vi "FlyWheelSim_GetCurrentDrawAmps.vi"(11 "FlyWheelSim":T1 {"GearBox"."Jr_KgM2" format="%13.5p"; "GearBox"."L_H" format="%13.5p"; "GearBox"."Kt_NMPerAmp" format="%13.5p"; "GearBox"."KvINV_RadPerSecPerVolt" format="%13.5p"; "GearBox"."R_Ohms" format="%13.5p"; "GearBox"."FreeSpeed_RadPerSec" format="%13.5p"; "GearBox"."FreeCurrent_Amps" format="%13.5p"; "GearBox"."StallCurrent_Amps" format="%13.5p"; "GearBox"."StallTorque_NM" format="%13.5p"; "GearBox"."nominalVoltage_Volts" format="%13.5p"}) -> (3 "Current_Amps":dbl)   [LabVIEW 2019, in "Trajectory_Library.lvlib"]
doc: "Returns the flywheel current draw.\n\nInputs:\n - FlyWheelSim -- Data cluster\n \nOutputs:\n - Current_Amps -- The flywheel current draw. (Amps)"
uses:
  Trajectory_Library.lvlib
  FLYWHEEL_SIM.ctl
  LINEAR_SYSTEM_SIM.ctl
  LINEAR_SYSTEM.ctl
  <vilib>/Analysis/Matrix/Datatypes/RealMatrix.ctl
  DCMOTOR.CTL
  <vilib>/Analysis/Matrix/NI_Matrix.lvlib
panel:
  # "<States, 1>"
  # "<Outputs, 1>"
  # "<Inputs, 1>"
  # "<Outputs, 1>"
  # "<States,States>"
  # "<States,Inputs>"
  # "<Outputs,States>"
  # "<Outputs,Inputs>"
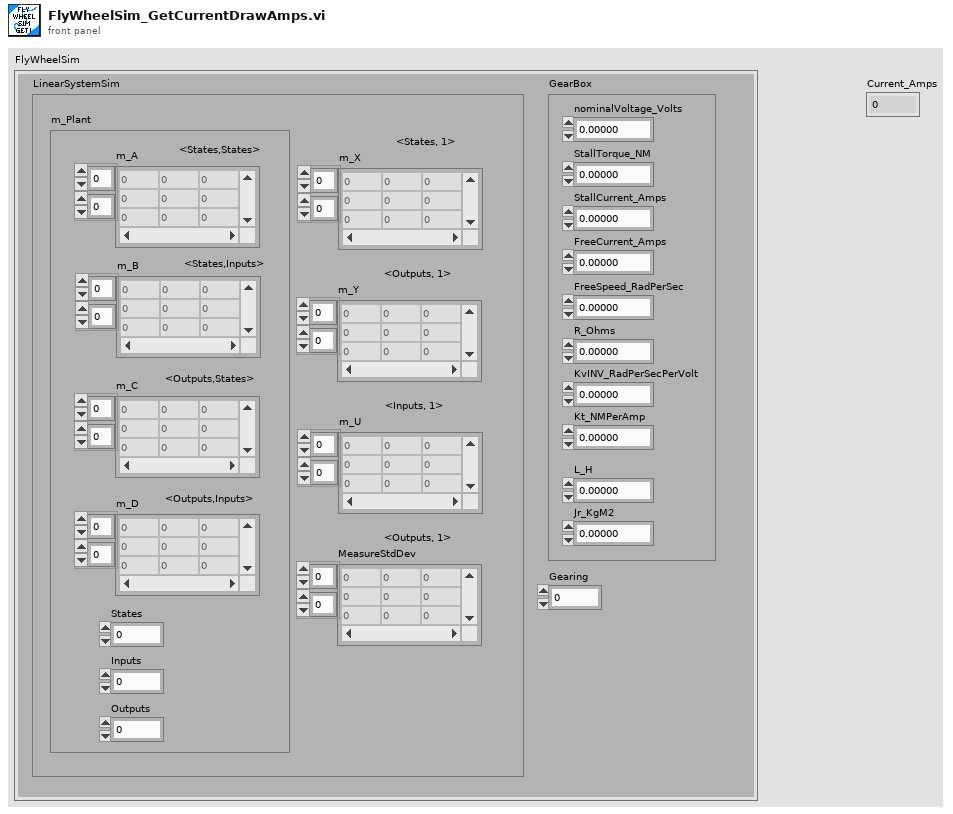
[diagram p1: front panel]
types:
  T1 = typedef "Trajectory_Library.lvlib/FLYWHEEL_SIM.ctl" = cluster{"LinearSystemSim":T2, "GearBox":T5, "Gearing":dbl}
  T2 = typedef "Trajectory_Library.lvlib/LINEAR_SYSTEM_SIM.ctl" = cluster{"m_Plant":T3, "m_X":T4, "m_Y":T4, "m_U":T4, "MeasureStdDev":T4}
  T3 = typedef "Trajectory_Library.lvlib/LINEAR_SYSTEM.ctl" = cluster{"m_A":T4, "m_B":T4, "m_C":T4, "m_D":T4, "States":i32, "Inputs":i32, "Outputs":i32}
  T4 = typedef "NI_Matrix.lvlib/RealMatrix.ctl" = dbl[][]
  T5 = typedef "Trajectory_Library.lvlib/DCMOTOR.CTL" = cluster{"nominalVoltage_Volts":dbl, "StallTorque_NM":dbl, "StallCurrent_Amps":dbl, "FreeCurrent_Amps":dbl, "FreeSpeed_RadPerSec":dbl, "R_Ohms":dbl, "KvINV_RadPerSecPerVolt":dbl, "Kt_NMPerAmp":dbl, "L_H":dbl, "Jr_KgM2":dbl}
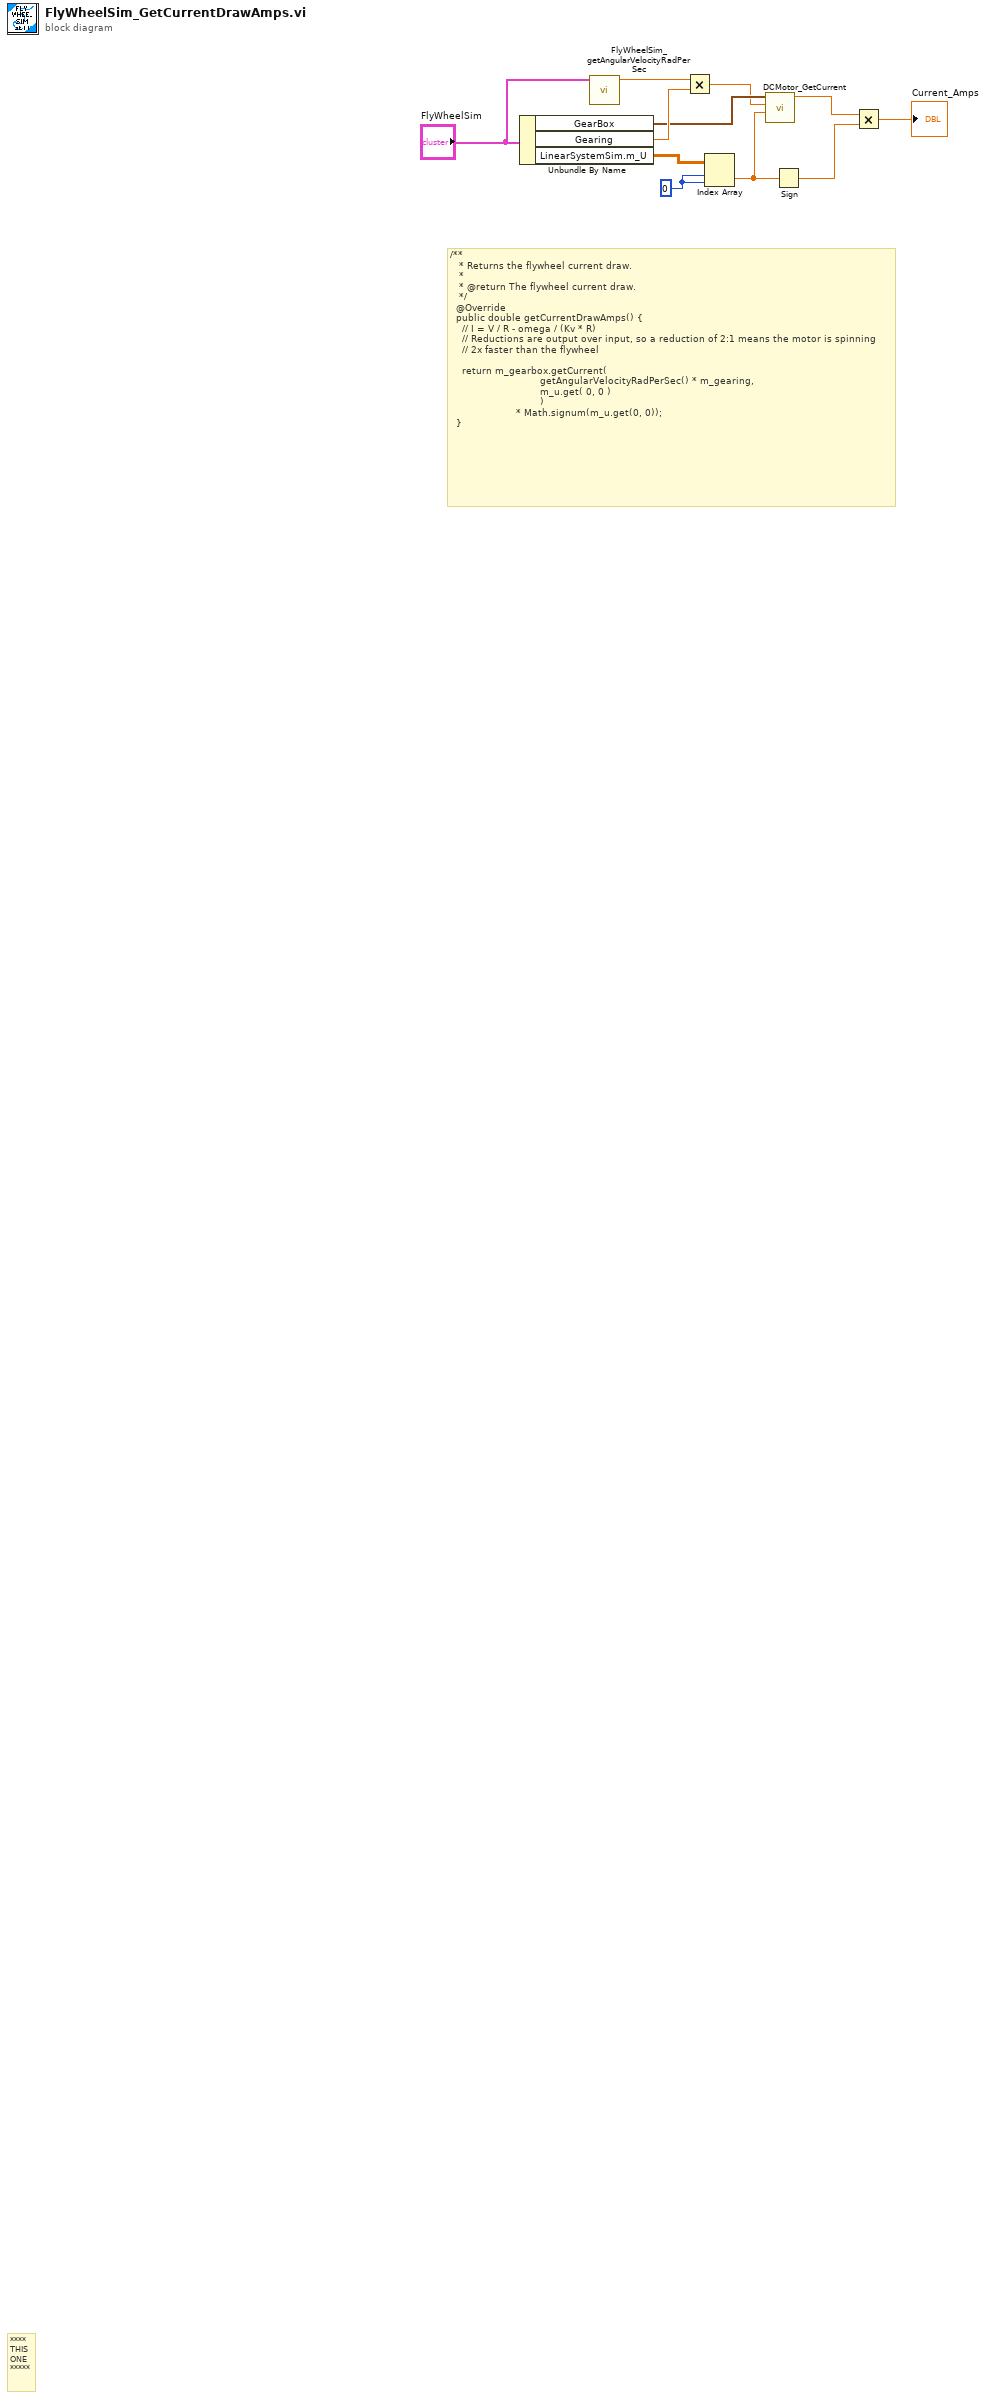
[diagram p0: block diagram]
diagram:
  w5 = 0 ("index (row)")
  # "/**\n   * Returns the flywheel current draw.\n   *\n   * @return The flywheel current draw.\n   */\n  @Override\n  public double getCurrentDrawAmps() {\n    // I = V / R - omega / (Kv * R)\n    // Reductions are output over input, so a reduction of 2:1 means the motor is spinning\n    // 2x faster than the flywheel\n\n    return m_gearbox.getCurrent(\n                              getAngularVelocityRadPerSec() * m_gearing, \n                              m_u.get( 0, 0 ) \n                              )\n                      * Math.signum(m_u.get(0, 0));\n  }"
  # "****\nTHIS\nONE\n*****"
  n1 = Unbundle By Name("FlyWheelSim") -> ("GearBox"=w8:T5, "Gearing"=w9:dbl, "LinearSystemSim.m_U"=w6:T4)
  n2 = call "FlyWheelSim_getAngularVelocityRadPerSec.vi"("FlyWheelSim"="FlyWheelSim") -> ("Velocity_RadPerSec"=w10:dbl)  [unwired: 10 in]
  n3 = Multiply(x=w10, y=w9) -> (x*y=w7:dbl)
  n4 = Index Array(array=w6, index (row)=w5, index (col)=w5) -> (element=w4:dbl)
  n5 = call "DCMotor_GetCurrent.vi"("VoltageInput_Volts"=w4, "Speed_RadPerSec"=w7, "DCMOTOR"=w8) -> ("Current_Amps"=w3:dbl)  [unwired: 8 in]
  n6 = Sign(1:w4) -> (0:w2:dbl)
  n7 = Multiply(x=w3, y=w2) -> (x*y=→"Current_Amps":dbl)
